vi "Read Valve Capillary Line State.vi"(7 "timeout in ms (-1)":i32, 8 "error in (no error)":errorcluster, 11 "Capillary Line in":refnum<class "Capillary Line.lvclass">) -> (0 "error out":errorcluster, 1 "timed out?":bool, 2 "Open?":bool, 3 "Capillary Line out":refnum<class "Capillary Line.lvclass">, 4 "Valve Capillary Line StateQ":refnum<queue>)   [LabVIEW 2015, in "cRIO-Carbondioxide.lvlib" / "CO2-Actor.lvlib" / "Capillary Line.lvclass"]
uses:
  Capillary Line.lvclass
  Capillary Line.lvclass/Capillary Line.ctl
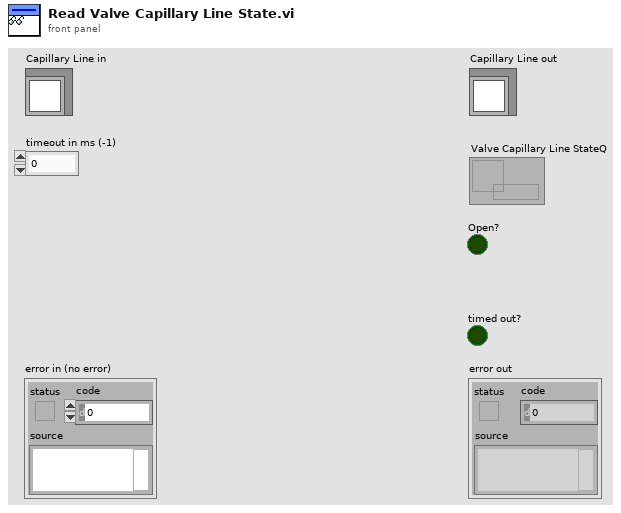
[diagram p1: front panel]
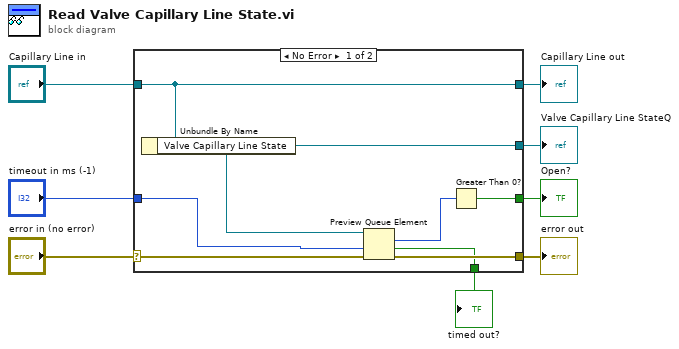
[diagram p0: block diagram]
diagram:
  n1 = case shown="No Error" "error in (no error)" {
    selector: "error in (no error)" -> [w15 w17]
    tunnel: [w14 w17] -> w7
    tunnel: [w16 w18] -> w5
    tunnel: "Capillary Line in" -> [w16 w18]
    tunnel: [w13 _] -> w4
    tunnel: [w9 _] -> w3
    tunnel: "timeout in ms (-1)" -> [w11 _]
    tunnel: [w10 _] -> w1
    frame No Error {
      n2 = Unbundle By Name(w16) -> ("Valve Capillary Line State"=w13:refnum<queue>)
      n3 = Preview Queue Element(queue=w13, timeout in ms (-1)=w11, error in (no error)=w15) -> (element=w12:u16, timed out?=w10:bool, error out=w14:errorcluster)  [unwired: 1 out]
      n4 = Greater Than 0?(x=w12) -> (x > 0?=w9:bool)
    }
    frame Error {
    }
  }
  "error out" <- w7
  "Capillary Line out" <- w5
  "Valve Capillary Line StateQ" <- w4
  "Open?" <- w3
  "timed out?" <- w1
